vi "Set Message Type.vi"(8 "error in":errorcluster, 10 "message type":T1, 11 "message in":T2 format="%.0x") -> (0 "error out":errorcluster, 3 "message out":T2 format="%.0x")   [LabVIEW 2020, in "AIM MIL-STD-1553 Scripting.lvlib"]
doc: "Reads the <b>description</b> field of the input <b>Ballard MIL-STD 1553 custom device</b>."
uses:
  AIM MIL-STD-1553 Scripting.lvlib
  Constants.vi
  <vilib>/NI VeriStand/Custom Device API/Custom Device API.lvlib
  <vilib>/NI VeriStand/Custom Device API/Set Item Property (String).vi
  <vilib>/NI VeriStand/Custom Device API/Custom Device Item Ref.ctl
  Shared/Message Type.ctl
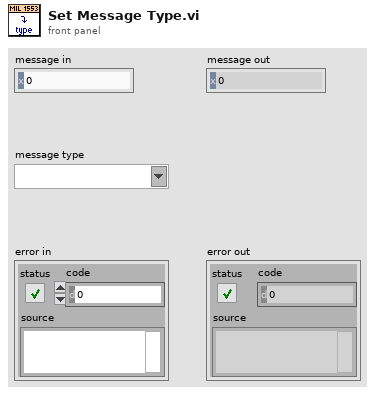
[diagram p1: front panel]
types:
  T1 = typedef "Message Type.ctl" = string
  T2 = typedef "Custom Device API.lvlib/Custom Device Item Ref.ctl" = u64
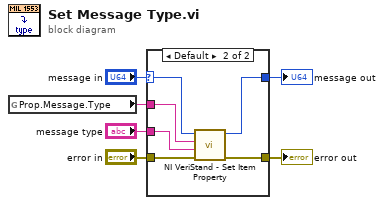
[diagram p0: block diagram]
diagram:
  n1 = global read "Constants.vi" "Prop.Message.Type"() -> (w2:string)
  n2 = case shown="Default" "message in" {
    selector: "message in" -> [w8 w14]
    tunnel: [w8 w13] -> w5
    tunnel: "error in" -> [w7 w12]
    tunnel: [w7 w11] -> w3
    tunnel: w2 -> [_ w10]
    tunnel: "message type" -> [_ w9]
    frame 0, -1 {
    }
    frame Default {
      n3 = call-poly <vilib>:"NI VeriStand - Set Item Property.vi"("error in (no error)"=w12, "Value"=w9, "Property Name"=w10, "Item Ref in"=w14) -> ("error out"=w11:errorcluster, "Item Ref out"=w13:T2)  [unwired: 5 in, 1 out]
    }
  }
  "message out" <- w5
  "error out" <- w3
